vi "SetMenu.vi"(8 "error in (no error)":errorcluster, 10 "menu":picture, 11 "menu in":refnum<class "menu.lvclass">) -> (0 "error out":errorcluster, 3 "menu out":refnum<class "menu.lvclass">)   [LabVIEW 2009, in "menu.lvclass"]
uses:
  menu.lvclass
  menu.lvclass/menu.ctl
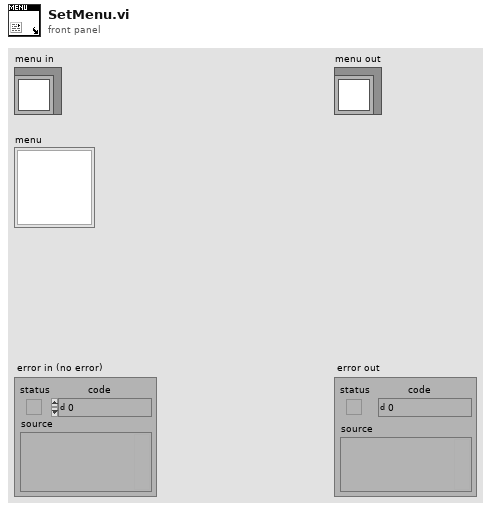
[diagram p1: front panel]
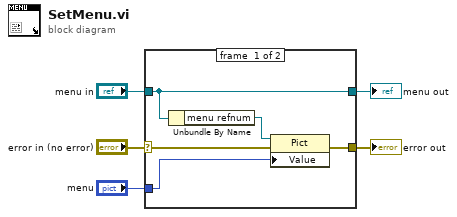
[diagram p0: block diagram]
diagram:
  n1 = case shown="No Error" "error in (no error)" {
    selector: "error in (no error)" -> [w10 w12]
    tunnel: [w9 w12] -> w2
    tunnel: [w8 w11] -> w4
    tunnel: "menu in" -> [w8 w11]
    tunnel: "menu" -> [w6 _]
    frame #0 {
      n2 = Unbundle By Name(w8) -> ("menu refnum"=w7:refnum<vi>)
      n3 = property class="Pict"(reference=w7, error in=w10, "Value"=w6) -> (error out=w9:errorcluster)  [unwired: 1 out]
    }
    frame #1 {
    }
  }
  "menu out" <- w4
  "error out" <- w2
